vi "Main.vi"(11 "Module Admin":refnum<class "Delacor_lib_QMH_Cloneable Module Admin.lvclass">) -> ()   [LabVIEW 2023, in "VoltageDataAquisition.lvlib"]
doc: "This template is based off of the Queued Message Handler design pattern and the Queued Message Handler project template that ships with LabVIEW.\n\nThe main difference is that the queue is private to this module and communication between modules is performed via Broadcast and Request events.\n\nRequest events are wrapped in public API methods and are handled in the Event Handling Loop (EHL) of this VI. Any module can register for Broadcast events sent by this module. The EHL generates messages based on user interface actions.\n\nThe Message Handling Loop (MHL) processes messages generated by the EHL, or by other messages. The messages are string values, so new messages can be added easily to the Message Cases case structure in the MHL. Each message cluster can also provide an optional value for Message Data, which is a variant that can be converted to whatever message-specific data is required.\n_____\nBased on DQMH Project Template 7.0.1.1316."
uses:
  VoltageDataAquisition.lvlib
  <vilib>/Delacor/Delacor QMH/Libraries/Cloneable Module Admin_class/Delacor_lib_QMH_Cloneable Module Admin.lvclass
  Module Data--cluster.ctl
  <vilib>/Delacor/Delacor QMH/Libraries/Message Queue_class/Delacor_lib_QMH_Message Queue.lvclass/Delacor_lib_QMH_Message Queue.ctl
  <vilib>/Delacor/Delacor QMH/Libraries/Cloneable Module Admin_class/Delacor_lib_QMH_Cloneable Module Admin.lvclass/Delacor_lib_QMH_Cloneable Module Admin.ctl
  Stop Argument--cluster.ctl
  <vilib>/Delacor/Delacor QMH/Libraries/Module Admin_class/Delacor_lib_QMH_Module Admin.lvclass/Delacor_lib_QMH_Module Admin.ctl
  DataRead Argument--cluster.ctl
  CreatDAQ Argument--cluster.ctl
  StopDAQ Argument--cluster.ctl
  <vilib>/Utility/miscctls.llb/LVPointTypeDef.ctl
  <vilib>/Delacor/Delacor QMH/Libraries/Message Queue_class/Delacor_lib_QMH_Enqueue Message (Single).vi
  <vilib>/Delacor/Delacor QMH/Libraries/Cloneable Module Admin_class/Delacor_lib_QMH_Get Module ID.vi
  <vilib>/Delacor/Delacor QMH/Libraries/Module Admin_class/Delacor_lib_QMH_Get External Launch.vi
  <vilib>/Delacor/Delacor QMH/Libraries/Message Queue_class/Delacor_lib_QMH_Message Queue.lvclass
  <vilib>/Analysis/NI_AALBase.lvlib
panel:
  out "Stop?":bool
  out "웨이브폼 그래프":dbl[](graph)
  out "error out":errorcluster
  out "Status":string
  in  "Simulate EHL Error":bool
  in  "Simulate MHL Error":bool
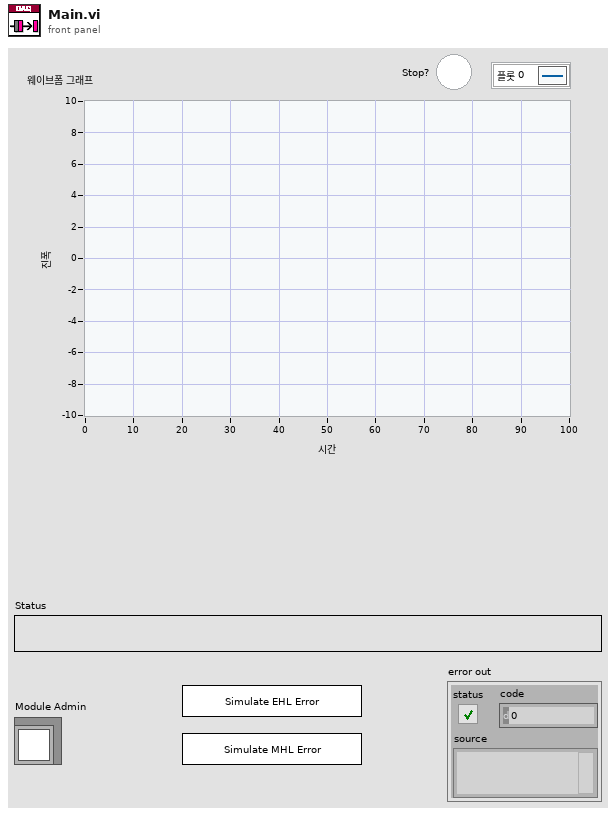
[diagram p1: front panel]
types:
  T1 = typedef "VoltageDataAquisition.lvlib/Request Events--cluster.ctl" = cluster{"Stop Module":refnum<user-event>, "Show Panel":refnum<user-event>, "Hide Panel":refnum<user-event>, "Show Diagram":refnum<user-event>, "Get Module Execution Status":refnum<user-event>, "DataRead":refnum<user-event>, "CreatDAQ":refnum<user-event>, "StopDAQ":refnum<user-event>}
  T2 = typedef "VoltageDataAquisition.lvlib/Module Data--cluster.ctl" = cluster{"Status":string, "웨이브폼 그래프":dbl[]}
  T3 = enum32{"invalid lock state", "Not Locked", "Locked (No Password)", "Password-protected"}
  T4 = typedef "VoltageDataAquisition.lvlib/Stop Argument--cluster.ctl" = cluster{"Module ID":i32, "Origin":string, "Exit via Stop Module Req?":bool, "Wait for Module to stop?":bool}
  T5 = typedef "VoltageDataAquisition.lvlib/DataRead Argument--cluster.ctl" = cluster{"Module ID":i32, "불리언":bool}
  T6 = typedef "VoltageDataAquisition.lvlib/CreatDAQ Argument--cluster.ctl" = cluster{"Module ID":i32, "불리언":bool}
  T7 = typedef "VoltageDataAquisition.lvlib/StopDAQ Argument--cluster.ctl" = cluster{"Module ID":i32, "불리언":bool}
  T8 = typedef "LVPointTypeDef.ctl" = cluster{"Horizontal":i16, "Vertical":i16}
  T9 = enum32{"Invalid", "Standard", "Closed", "Hidden", "Minimized", "Maximized"}
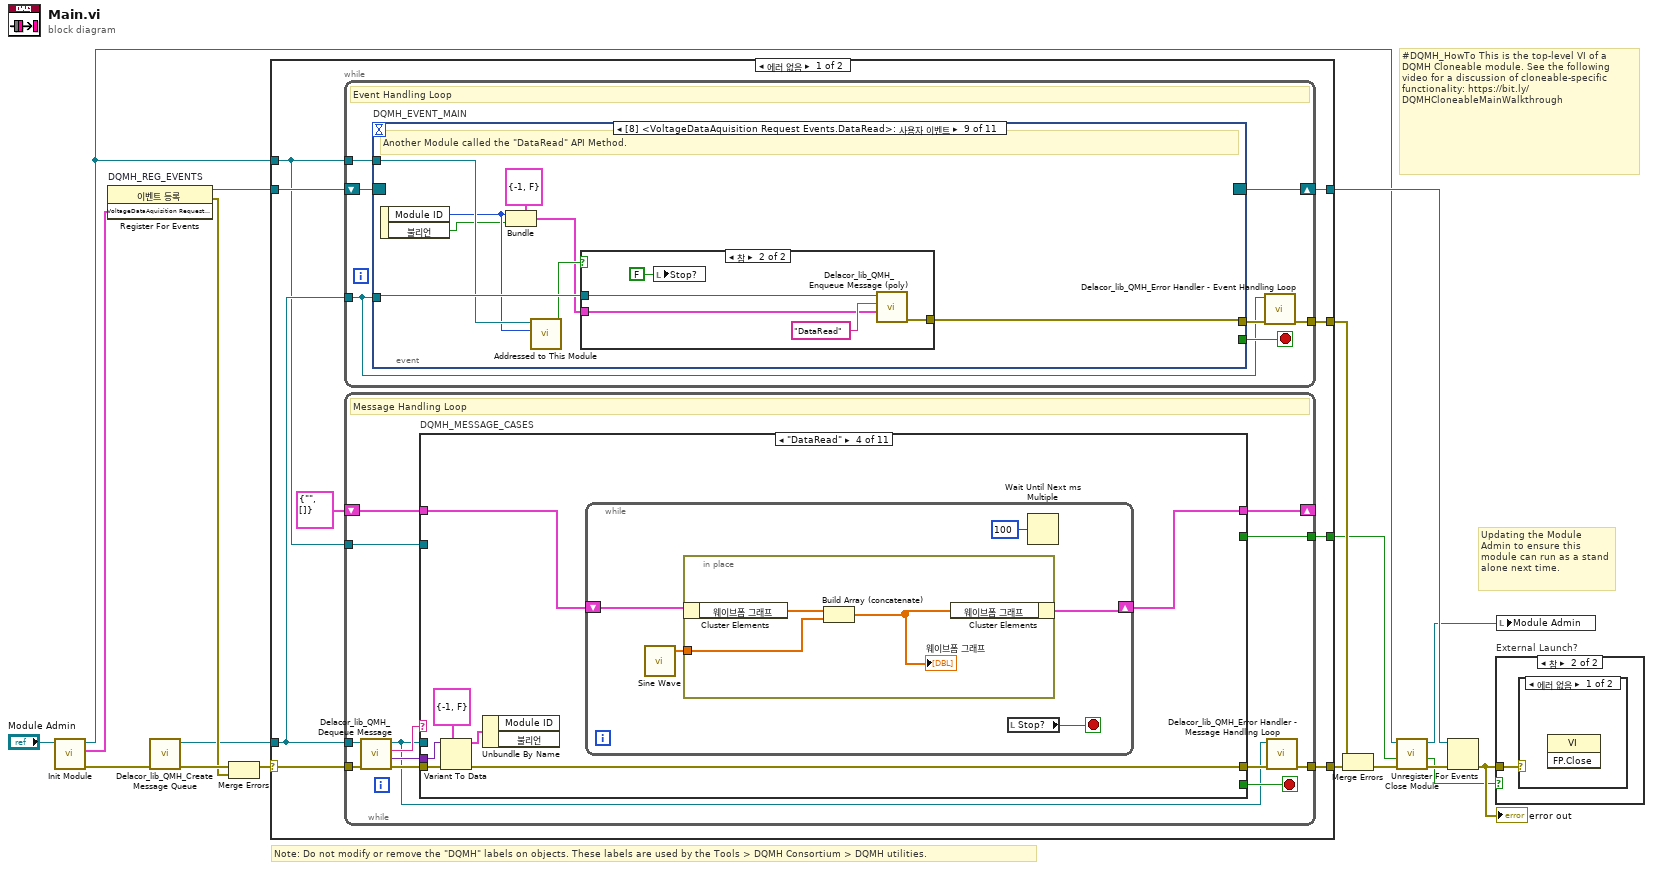
[diagram p0: block diagram]
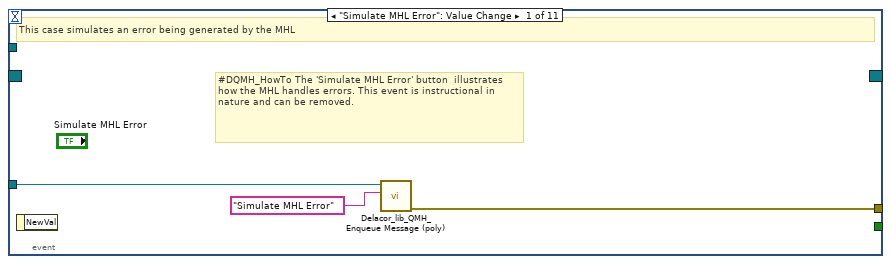
[diagram p2: hidden frame]
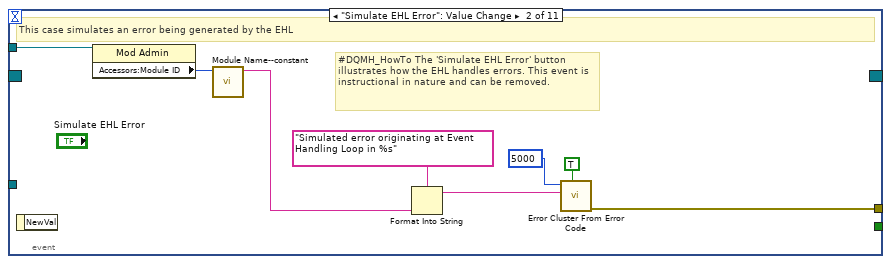
[diagram p3: hidden frame]
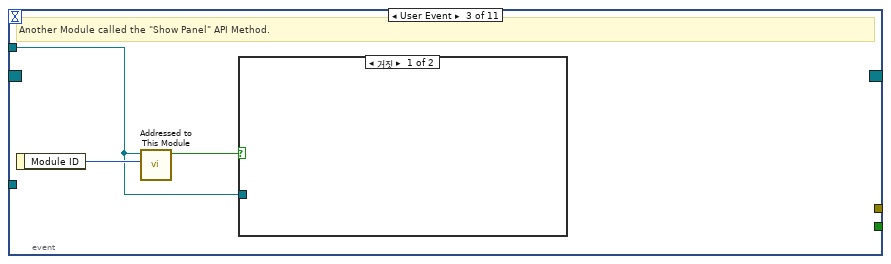
[diagram p4: hidden frame]
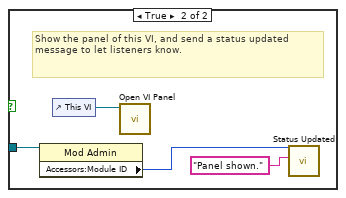
[diagram p5: hidden frame]
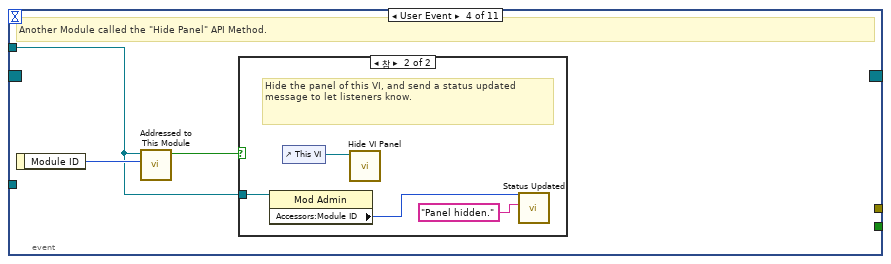
[diagram p6: hidden frame]
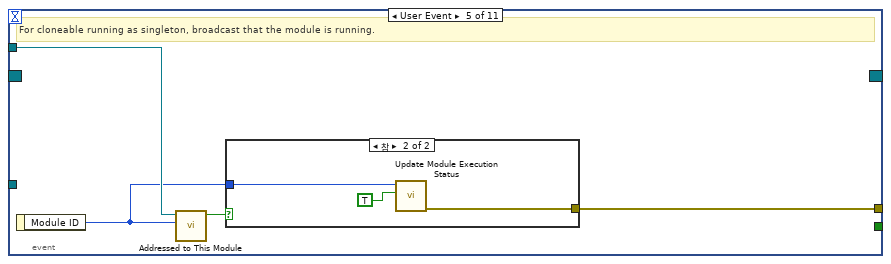
[diagram p8: hidden frame]
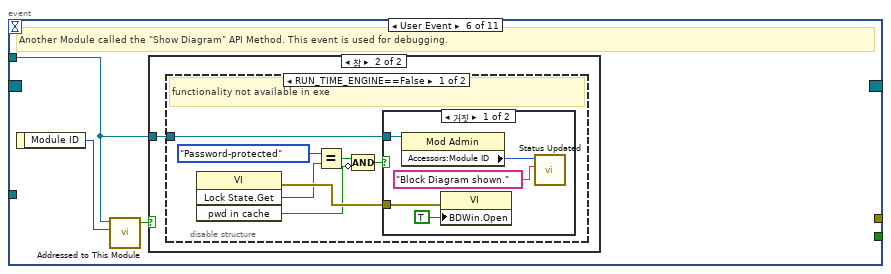
[diagram p10: hidden frame]
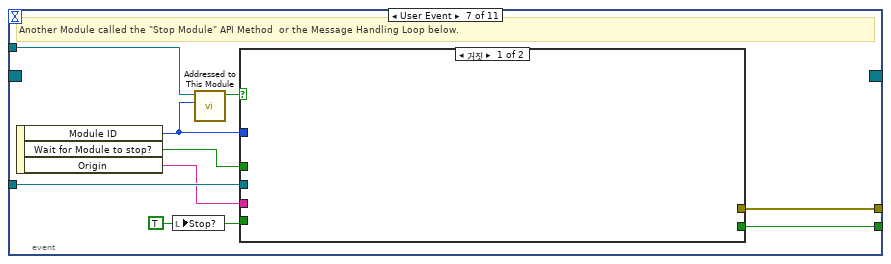
[diagram p14: hidden frame]
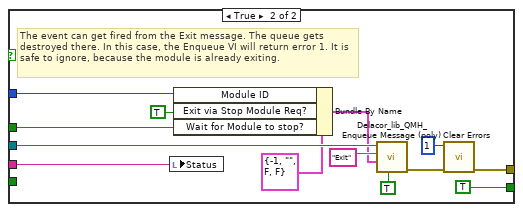
[diagram p15: hidden frame]
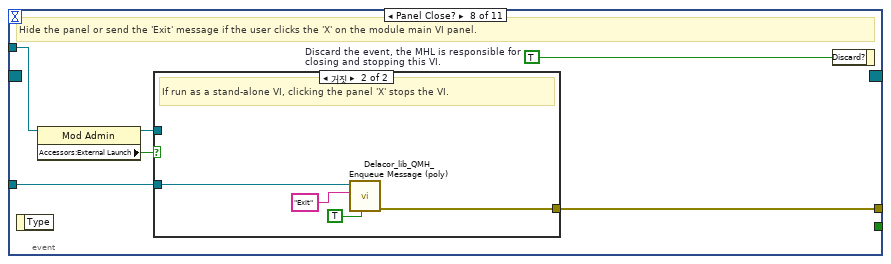
[diagram p16: hidden frame]
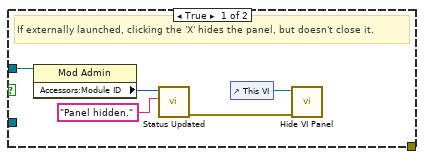
[diagram p17: hidden frame]
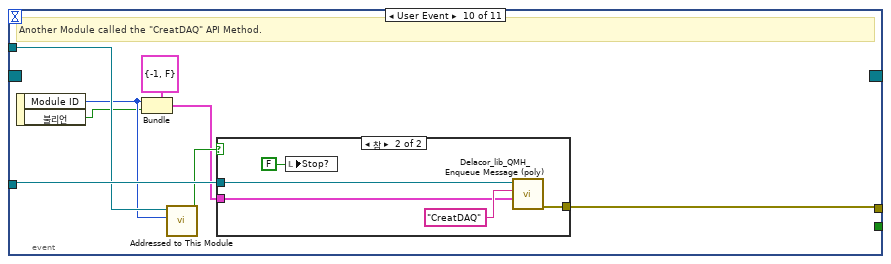
[diagram p19: hidden frame]
diagram:
  # "#DQMH_HowTo This is the top-level VI of a DQMH Cloneable module. See the following video for a discussion of cloneable-specific functionality: https://bit.ly/DQMHCloneableMainWalkthrough"
  # "Note: Do not modify or remove the \"DQMH\" labels on objects. These labels are used by the Tools > DQMH Consortium > DQMH utilities."
  # "Updating the Module Admin to ensure this module can run as a stand alone next time."
  n1 = call "Init Module.vi"("Cloneable Module Admin in"="Module Admin") -> ("error out"=w15:errorcluster, "VoltageDataAquisition Request Events"=w7:T1, "Cloneable Module Admin out"=w4:refnum<class "Delacor_lib_QMH_Cloneable Module Admin.lvclass">)  [unwired: 8 in]
  n2 = register-events "DQMH_REG_EVENTS"(w7) -> (reference out=w8:refnum<event-registration>, error out=w10:errorcluster)  [unwired: 2 in]
  n3 = call <vilib>:"Delacor_lib_QMH_Create Message Queue.vi"("error in"=w15) -> ("error out"=w12:errorcluster, "Message Queue"=w6:refnum<class "Delacor_lib_QMH_Message Queue.lvclass">)  [unwired: 9 in]
  n4 = Merge Errors(w12, w10) -> (w11:errorcluster)
  n5 = case shown="에러 없음" w11 {
    selector: w11 -> [w25 w295]
    tunnel: [w27 w294] -> w16
    tunnel: [w24 w293] -> w9
    tunnel: w8 -> [w22 w293]
    tunnel: w6 -> [w21 w286]
    tunnel: [w26 _] -> w17
    tunnel: w4 -> [w20 w289]
    tunnel: [w19 _] -> w2
    frame No Error {
      n6 = while {
        tunnel: w21 -> [w28]
        shift-right: [w31] -> w24
        shift-left: w22 -> [w32]
        tunnel: [w33] -> w26
        tunnel: w20 -> [w29]
        stop <- w30 stop-if-true
        # "Event Handling Loop"
        n7 = event "DQMH_EVENT_MAIN" shown="[8] <VoltageDataAquisition Request Events.DataRead>: 사용자 이벤트" {
          selector: w32 -> [_ _ _ _ _ _ _ _ _ _ _]
          dyn-events: [_ _ _ _ _ _ _ _ _ _ _] -> w31
          timeout: _ -> [_ _ _ _ _ _ _ _ _ _ _]
          tunnel: [_ _ _ _ _ _ w87 _ _ _ _] -> w30
          tunnel: w28 -> [w36 _ _ _ _ _ w90 w107 w127 w140 w153]
          tunnel: [w37 w45 _ _ w63 _ w91 w110 w120 w133 w146] -> w34
          tunnel: w29 -> [_ w44 w46 w53 w61 w67 w89 w108 w125 w138 w151]
          event "Simulate MHL Error": Value Change {
            # "#DQMH_HowTo The 'Simulate MHL Error' button  illustrates how the MHL handles errors. This event is instructional in nature and can be removed."
            # "This case simulates an error being generated by the MHL"
            n8 = event-data() -> ()  [unwired: 1 in, 1 out]
            n9 = call-poly <vilib>:"Delacor_lib_QMH_Enqueue Message (poly).vi"("Message"="Simulate MHL Error", "Message Queue in"=w36) -> ("error out"=w37:errorcluster)  [unwired: 8 in, 1 out]
          }
          event "Simulate EHL Error": Value Change {
            # "#DQMH_HowTo The 'Simulate EHL Error' button  illustrates how the EHL handles errors. This event is instructional in nature and can be removed."
            # "This case simulates an error being generated by the EHL"
            n10 = event-data() -> ()  [unwired: 1 in, 1 out]
            n11 = property on="Property Node" class="Mod Admin"(reference=w44) -> ("Accessors:Module ID"=w43:i32)  [unwired: 1 in, 2 out]
            n12 = call "Module Name--constant.vi"("Module ID"=w43) -> ("Module Name"=w38:string)  [unwired: 10 in]
            n13 = Format Into String(format string="Simulated error originating at Event Handling Loop in %s", w38) -> (resulting string=w41:string)  [unwired: 2 in, 1 out]
            n14 = call <vilib>:"Error Cluster From Error Code.vi"("show call chain? (False)"=TRUE, "error message (\"\")"=w41, "error code (0)"=5000) -> ("error out"=w45:errorcluster)  [unwired: 6 in]
          }
          event User Event {
            # "Another Module called the \"Show Panel\" API Method."
            n15 = event-data() -> ("Module ID"=w47:i32)  [unwired: 1 in]
            n16 = call "Addressed to This Module.vi"("Module ID from Argument"=w47, "Module Admin"=w46) -> ("Addressed to this instance?"=w48:bool)  [unwired: 8 in, 1 out]
            n17 = case shown="거짓" w48 {
              tunnel: w46 -> [_ w50]
              frame False {
              }
              frame True {
                # "Show the panel of this VI, and send a status updated message to let listeners know."
                n18 = property on="Property Node" class="Mod Admin"(reference=w50) -> ("Accessors:Module ID"=w49:i32)  [unwired: 1 in, 2 out]
                n19 = control-ref of="This VI"() -> (w52:refnum<vi>)
                n20 = call "Open VI Panel.vi"("VI"=w52) -> ()  [unwired: 10 in, 1 out]
                n21 = call "Status Updated.vi"("Status"="Panel shown." ("format string"), "Module ID"=w49) -> ()  [unwired: 9 in, 1 out]
              }
            }
          }
          event User Event {
            # "Another Module called the \"Hide Panel\" API Method."
            n22 = event-data() -> ("Module ID"=w54:i32)  [unwired: 1 in]
            n23 = call "Addressed to This Module.vi"("Module ID from Argument"=w54, "Module Admin"=w53) -> ("Addressed to this instance?"=w55:bool)  [unwired: 8 in, 1 out]
            n24 = case shown="참" w55 {
              tunnel: w53 -> [_ w57]
              frame False {
              }
              frame True {
                # "Hide the panel of this VI, and send a status updated message to let listeners know."
                n25 = property on="Property Node" class="Mod Admin"(reference=w57) -> ("Accessors:Module ID"=w56:i32)  [unwired: 1 in, 2 out]
                n26 = control-ref of="This VI"() -> (w59:refnum<vi>)
                n27 = call "Hide VI Panel.vi"("VI"=w59) -> ()  [unwired: 10 in, 1 out]
                n28 = call "Status Updated.vi"("Status"="Panel hidden." ("format string"), "Module ID"=w56) -> ()  [unwired: 9 in, 1 out]
              }
            }
          }
          event User Event {
            # "For cloneable running as singleton, broadcast that the module is running."
            n29 = event-data() -> ("Module ID"=w60:i32)  [unwired: 1 in]
            n30 = call "Addressed to This Module.vi"("Module ID from Argument"=w60, "Module Admin"=w61) -> ("Addressed to this instance?"=w62:bool)  [unwired: 8 in, 1 out]
            n31 = case shown="참" w62 {
              tunnel: [_ w66] -> w63
              tunnel: w60 -> [_ w65]
              frame False {
              }
              frame True {
                n32 = call "Update Module Execution Status.vi"("Running?"=TRUE, "Module ID"=w65) -> ("error out"=w66:errorcluster)  [unwired: 9 in]
              }
            }
          }
          event User Event {
            # "Another Module called the \"Show Diagram\" API Method. This event is used for debugging."
            n33 = event-data() -> ("Module ID"=w68:i32)  [unwired: 1 in]
            n34 = call "Addressed to This Module.vi"("Module ID from Argument"=w68, "Module Admin"=w67) -> ("Addressed to this instance?"=w69:bool)  [unwired: 8 in, 1 out]
            n35 = case shown="참" w69 {
              tunnel: w67 -> [_ w70]
              frame False {
              }
              frame True {
                n36 = disable-structure shown="RUN_TIME_ENGINE==False" {
                  disable-tunnel: w70 -> [w71 _]
                  frame condition #0 (active) {
                    # "functionality not available in exe"
                    n37 = invoke on="Invoke Node" class="VI" method="Lock State.Get"() -> (error out=w77:errorcluster, "Get Lock State"=w76:T3, "pwd in cache"=w73:bool)  [unwired: 4 in, 1 out]
                    n38 = Equal?(x=T3."Password-protected", y=w76) -> (x = y?=w74:bool)
                    n39 = Compound Arithmetic op=AND(w74, invert w73) -> (w72:bool)
                    n40 = case shown="거짓" w72 {
                      tunnel: w77 -> [w82 _]
                      tunnel: w71 -> [w79 _]
                      frame False {
                        n41 = property on="Property Node" class="Mod Admin"(reference=w79) -> ("Accessors:Module ID"=w78:i32)  [unwired: 1 in, 2 out]
                        n42 = property on="Property Node" class="VI"(error in=w82, "BDWin.Open"=TRUE ("Block Diagram Window:Open")) -> ()  [unwired: 1 in, 2 out]
                        n43 = call "Status Updated.vi"("Status"="Block Diagram shown." ("format string"), "Module ID"=w78) -> ()  [unwired: 9 in, 1 out]
                      }
                      frame True {
                        # "Password-protected VI, and the password is not in the cache. Do not show the diagram."
                      }
                    }
                  }
                  frame condition #1 {
                  }
                }
              }
            }
          }
          event User Event {
            w83 = TRUE ("Stop?")
            # "Another Module called the \"Stop Module\" API Method  or the Message Handling Loop below."
            n44 = event-data() -> ("Module ID"=w85:i32, "Wait for Module to stop?"=w86:bool, "Origin"=w84:string)  [unwired: 1 in]
            n45 = local write "Stop?"(w83) -> ()
            n46 = call "Addressed to This Module.vi"("Module ID from Argument"=w85, "Module Admin"=w89) -> ("Addressed to this instance?"=w88:bool)  [unwired: 8 in, 1 out]
            n47 = case shown="거짓" w88 {
              tunnel: [_ w103] -> w91
              tunnel: w90 -> [_ w99]
              tunnel: [_ TRUE] -> w87
              tunnel: w86 -> [_ w92]
              tunnel: w85 -> [_ w96]
              tunnel: w84 -> [_ w93]
              tunnel: w83 -> [_ _]
              frame False {
              }
              frame True {
                # "The event can get fired from the Exit message. The queue gets destroyed there. In this case, the Enqueue VI will return error 1. It is safe to ignore, because the module is already exiting."
                n48 = local write "Status"(w93) -> ()
                n49 = Bundle By Name(cluster=T4 {"Module ID"=-1, "Origin"="", "Exit via Stop Module Req?"=FALSE, "Wait for Module to stop?"=FALSE} ("Stop Argument"), "Module ID"=w96, "Exit via Stop Module Req?"=TRUE, "Wait for Module to stop?"=w92) -> (w94:T4)
                n50 = call-poly <vilib>:"Delacor_lib_QMH_Enqueue Message (poly).vi"("Priority Message? (F)"=TRUE, "Message Data"=w94, "Message"="Exit", "Message Queue in"=w99) -> ("error out"=w104:errorcluster)  [unwired: 6 in, 1 out]
                n51 = call <vilib>:"Clear Errors.vi"("error in (no error)"=w104, "specific error code to clear (0: all)"=1) -> ("error out"=w103:errorcluster)  [unwired: 4 in, 1 out]
              }
            }
          }
          event Panel Close? {
            w109 = TRUE  # Discard the event, the MHL is responsible for closing and stopping this VI.
            # "Hide the panel or send the 'Exit' message if the user clicks the 'X' on the module main VI panel."
            n52 = event-data() -> ()  [unwired: 1 in, 1 out]
            n53 = property on="Property Node" class="Mod Admin"(reference=w108) -> (reference out=w105:refnum<class "Delacor_lib_QMH_Cloneable Module Admin.lvclass">, "Accessors:External Launch"=w106:bool)  [unwired: 1 in, 1 out]
            n54 = case shown="거짓" w106 {
              tunnel: w107 -> [_ w118]
              tunnel: [_ w119] -> w110
              tunnel: w105 -> [w113 _]
              frame True {
                # "If externally launched, clicking the 'X' hides the panel, but doesn't close it."
                n55 = property on="Property Node" class="Mod Admin"(reference=w113) -> ("Accessors:Module ID"=w112:i32)  [unwired: 1 in, 2 out]
                n56 = call "Status Updated.vi"("Status"="Panel hidden." ("format string"), "Module ID"=w112) -> ("error out"=w111:errorcluster)  [unwired: 9 in]
                n57 = control-ref of="This VI"() -> (w115:refnum<vi>)
                n58 = call "Hide VI Panel.vi"("error in"=w111, "VI"=w115) -> ()  [unwired: 9 in, 1 out]
              }
              frame False {
                # "If run as a stand-alone VI, clicking the panel 'X' stops the VI."
                n59 = call-poly <vilib>:"Delacor_lib_QMH_Enqueue Message (poly).vi"("Priority Message? (F)"=TRUE, "Message"="Exit", "Message Queue in"=w118) -> ("error out"=w119:errorcluster)  [unwired: 7 in, 1 out]
              }
            }
            n60 = event-data ("Event Filter Node")("Discard?"=w109) -> ()  [unwired: 1 in, 1 out]
          }
          event User Event {
            # "Another Module called the \"DataRead\" API Method."
            n61 = event-data() -> ("Module ID"=w122:i32, "불리언"=w121:bool)  [unwired: 1 in]
            n62 = Bundle(cluster=T5 {"Module ID"=-1, "불리언"=FALSE} ("DataRead Argument"), "Module ID"=w122, "불리언"=w121) -> (w123:T5)
            n63 = call "Addressed to This Module.vi"("Module ID from Argument"=w122, "Module Admin"=w125) -> ("Addressed to this instance?"=w126:bool)  [unwired: 8 in, 1 out]
            n64 = case "케이스 구조" shown="참" w126 {
              tunnel: w127 -> [_ w132]
              tunnel: w123 -> [_ w130]
              tunnel: [_ w129] -> w120
              frame False {
              }
              frame True {
                n65 = local write "Stop?"(FALSE ("Stop?")) -> ()
                n66 = call-poly <vilib>:"Delacor_lib_QMH_Enqueue Message (poly).vi"("Message Data"=w130, "Message"="DataRead", "Message Queue in"=w132) -> ("error out"=w129:errorcluster)  [unwired: 7 in, 1 out]
              }
            }
          }
          event User Event {
            # "Another Module called the \"CreatDAQ\" API Method."
            n67 = event-data() -> ("Module ID"=w135:i32, "불리언"=w134:bool)  [unwired: 1 in]
            n68 = Bundle(cluster=T6 {"Module ID"=-1, "불리언"=FALSE} ("CreatDAQ Argument"), "Module ID"=w135, "불리언"=w134) -> (w136:T6)
            n69 = call "Addressed to This Module.vi"("Module ID from Argument"=w135, "Module Admin"=w138) -> ("Addressed to this instance?"=w139:bool)  [unwired: 8 in, 1 out]
            n70 = case "케이스 구조" shown="참" w139 {
              tunnel: w140 -> [_ w145]
              tunnel: w136 -> [_ w143]
              tunnel: [_ w142] -> w133
              frame False {
              }
              frame True {
                n71 = local write "Stop?"(FALSE ("Stop?")) -> ()
                n72 = call-poly <vilib>:"Delacor_lib_QMH_Enqueue Message (poly).vi"("Message Data"=w143, "Message"="CreatDAQ", "Message Queue in"=w145) -> ("error out"=w142:errorcluster)  [unwired: 7 in, 1 out]
              }
            }
          }
          event User Event {
            # "Another Module called the \"StopDAQ\" API Method."
            n73 = event-data() -> ("Module ID"=w148:i32, "불리언"=w147:bool)  [unwired: 1 in]
            n74 = Bundle(cluster=T7 {"Module ID"=-1, "불리언"=FALSE} ("StopDAQ Argument"), "Module ID"=w148, "불리언"=w147) -> (w149:T7)
            n75 = call "Addressed to This Module.vi"("Module ID from Argument"=w148, "Module Admin"=w151) -> ("Addressed to this instance?"=w152:bool)  [unwired: 8 in, 1 out]
            "Stop?" <- w152
            n76 = case "케이스 구조" shown="참" w152 {
              tunnel: w153 -> [_ w157]
              tunnel: w149 -> [_ w155]
              tunnel: [_ w154] -> w146
              frame False {
              }
              frame True {
                n77 = call-poly <vilib>:"Delacor_lib_QMH_Enqueue Message (poly).vi"("Message Data"=w155, "Message"="StopDAQ", "Message Queue in"=w157) -> ("error out"=w154:errorcluster)  [unwired: 7 in, 1 out]
              }
            }
          }
        }
        n78 = call-dynamic "Delacor_lib_QMH_Error Handler - Event Handling Loop.vi"("error in"=w34, "Message Queue in"=w28) -> ("dup error in"=w33:errorcluster)  [unwired: 8 in, 1 out]
      }
      n79 = while {
        tunnel: w21 -> [w158]
        shift-right: [w165] -> _
        shift-left: T2 {"Status"="", "웨이브폼 그래프"=[]} ("Data Cluster") -> [w166]
        tunnel: w25 -> [w169]
        tunnel: [w167] -> w27
        tunnel: w20 -> [w160]
        tunnel: [w159] -> w19
        stop <- w164 stop-if-true
        # "Message Handling Loop"
        n80 = call-dynamic "Delacor_lib_QMH_Dequeue Message.vi"("error in"=w169, "Message Queue in"=w158) -> ("error out"=w168:errorcluster, "Message Data"=w162:variant, "Message"=w163:string, "Message Queue out"=w161:refnum<class "Delacor_lib_QMH_Message Queue.lvclass">)  [unwired: 6 in]
        n81 = case "DQMH_MESSAGE_CASES" shown="\"DataRead\"" w163 {
          selector: w163 -> [_ _ _ _ _ _ _ _ _ _ w275]
          tunnel: w161 -> [_ _ _ _ _ _ _ w230 _ w267 _]
          tunnel: w168 -> [w189 w193 w200 w208 w222 w225 w227 w239 w256 w273 w284]
          tunnel: [w187 w193 w199 w207 w220 w224 w227 w235 w255 w268 w285] -> w170
          tunnel: w166 -> [w180 w192 w195 w203 w221 w223 w226 w234 w253 w266 w282]
          tunnel: [w179 w192 w194 w202 w221 w223 w226 w234 w253 w266 w282] -> w165
          tunnel: [_ _ _ _ _ _ _ _ _ w265 _] -> w164
          tunnel: w162 -> [_ _ w198 w206 w219 _ _ w233 _ w263 _]
          tunnel: w160 -> [w174 _ _ _ _ _ _ w232 w251 w258 w281]
          tunnel: [_ _ _ _ _ _ _ _ _ w261 _] -> w159
          frame "Initialize" {
            w171 = "Initial Message" ("Initial Message")
            # "#CodeNeeded - Initialize the appearance of the front panel."
            # "#CodeNeeded - Initialize your state data here."
            # "Initialize - Any operation that needs to be done before the module can receive messages. Synchronize Caller Events.vi will inform Start Module.vi that the module has launched and is ready to receive messages. Module Did Init.vi will broadcast that the module initialized."
            n82 = call "Synchronize Caller Events.vi"("error in"=w189, "Module Admin"=w174) -> ("error out"=w188:errorcluster, "Module Admin out"=w173:refnum<class "Delacor_lib_QMH_Cloneable Module Admin.lvclass">)  [unwired: 8 in]
            n83 = property on="Property Node" class="Mod Admin"(reference=w173) -> ("Accessors:Module ID"=w176:i32, "Accessors:External Launch"=w175:bool)  [unwired: 1 in, 2 out]
            n84 = call "Module Name--constant.vi"("Module ID"=w176) -> ("Module Name"=w184:string)  [unwired: 10 in]
            n85 = property on="Property Node" class="VI"("Front Panel.Title"=w184) -> (reference out=w186:refnum<vi>, error out=w191:errorcluster)  [unwired: 2 in]
            n86 = Select(t=T9."Hidden" ("State"), s=w175, f=T9."Standard" ("State")) -> (s? t:f=w181:T9)
            n87 = invoke on="Invoke Node" class="VI" method="FP.Open"(reference=w186, error in=w191, "State"=w181) -> (reference out=w185:refnum<vi>, error out=w190:errorcluster)  [unwired: 2 in, 3 out]
            n88 = call "Module Name--constant.vi"("Module ID"=w176) -> ("Module Name"=w177:string)  [unwired: 10 in]
            n89 = Bundle By Name(cluster=w180, "Status"=w171) -> (w179:T2)
            n90 = invoke on="Invoke Node" class="VI" method="FP.Center"(reference=w185, error in=w190) -> ()  [unwired: 1 in, 3 out]
            n91 = property on="Pane" class="Pane"("Origin"=T8 {"Horizontal"=0, "Vertical"=0}) -> ()  [unwired: 2 in, 2 out]
            n92 = call "Module Did Init.vi"("error in"=w188, "Initialized?"=TRUE, "Origin"=w177, "Module ID"=w176) -> ("error out"=w187:errorcluster)  [unwired: 7 in]
            "Status" <- w171
          }
          frame "---Module Specific---" {
            # "Separator -- The following cases handle messages specific to this Module."
          }
          frame "CreatDAQ" {
            n93 = Variant To Data(error in=w200, type=T6 {"Module ID"=-1, "불리언"=FALSE} ("CreatDAQ Argument"), Variant=w198) -> (data=w196:T6, error out=w199:errorcluster)
            n94 = Unbundle By Name(w196) -> ()  [unwired: 2 out]
            n95 = in-place {
              n96 = in-place-cluster #1(w195) -> ()  [unwired: 1 out]
              n97 = in-place-cluster #1("웨이브폼 그래프"=dbl[] [] ("웨이브폼 차트")) -> (w194:T2)
            }
          }
          frame "DataRead" {
            n98 = Variant To Data(error in=w208, type=T5 {"Module ID"=-1, "불리언"=FALSE} ("DataRead Argument"), Variant=w206) -> (data=w204:T5, error out=w207:errorcluster)
            n99 = Unbundle By Name(w204) -> ()  [unwired: 2 out]
            n100 = while {
              shift-right: [w212] -> w202
              shift-left: w203 -> [w213]
              stop <- w211 stop-if-true
              n101 = call <vilib>:"Sine Wave.vi"() -> ("sine wave"=w209:dbl[])  [unwired: 5 in, 2 out]
              n102 = in-place {
                in-place-border: w209 -> [w215]
                n103 = in-place-cluster #2(w213) -> ("웨이브폼 그래프"=w216:dbl[])
                n104 = Build Array (concatenate)(w216, w215) -> (w214:dbl[])
                "웨이브폼 그래프" <- w214
                n105 = in-place-cluster #2("웨이브폼 그래프"=w214) -> (w212:T2)
              }
              n106 = local read "Stop?"() -> (w211:bool)
              n107 = Wait Until Next ms Multiple(millisecond multiple=u32 100 ("ms 배수")) -> ()  [unwired: 1 out]
            }
          }
          frame "StopDAQ" {
            n108 = Variant To Data(error in=w222, type=T7 {"Module ID"=-1, "불리언"=FALSE} ("StopDAQ Argument"), Variant=w219) -> (data=w217:T7, error out=w220:errorcluster)
            n109 = Unbundle By Name(w217) -> ()  [unwired: 2 out]
          }
          frame "---Copy This Frame---" {
            # "Duplicate this frame when creating new messages.  Change this comment in the duplicated frame to describe this message."
            n110 = Merge Errors(w225) -> (w224:errorcluster)
          }
          frame "---Exit and Error Handling---" {
            # "Separator - the following cases handle errors and exit messages."
          }
          frame "Error" {
            # "#CodeRecommended - If the module is running in standalone mode (External Launch = FALSE), this code will pop up an error dialog and call the 'Exit' message if an error occurs. Add more fine-grained error management here."
            # "Error - Check the error message data and respond accordingly. This message is sent by the \"Error Handler\" VIs at the end of each loop in this application."
            n111 = property on="Property Node" class="Mod Admin"(reference=w232) -> ("Accessors:External Launch"=w231:bool, "Accessors:Module ID"=w229:i32)  [unwired: 1 in, 2 out]
            n112 = Variant To Data(error in=w239, type=errorcluster {"status"=FALSE, "code"=0, "source"=""} ("error constant"), Variant=w233) -> (data=w228:errorcluster, error out=w237:errorcluster)
            n113 = local write "error out"(w228) -> ()
            n114 = call "Error Reported.vi"("Error"=w228, "Module ID"=w229) -> ()  [unwired: 9 in, 1 out]
            n115 = case shown="거짓" w231 {
              tunnel: [w244 _] -> w236
              tunnel: w230 -> [w242 _]
              tunnel: w228 -> [w243 _]
              frame False {
                n116 = disable-structure shown="Default" {
                  disable-tunnel: w243 -> [w245 _]
                  frame condition #0 (active) {
                    # "If the module is running standalone, then pop up an error dialog and call the \"Exit\" message."
                    n117 = call <vilib>:"Simple Error Handler.vi"("error in (no error)"=w245) -> ()  [unwired: 4 in, 5 out]
                  }
                  frame condition #1 {
                    # "To prevent the Simple Error Handler VI from being loaded (e.g. when deploying to a Real-Time target), add the Conditional Disable Symbol \"DQMH_Disable_SEH\" to your project and set it to TRUE."
                  }
                }
                n118 = call-poly <vilib>:"Delacor_lib_QMH_Enqueue Message (poly).vi"("Priority Message? (F)"=TRUE, "Message"="Exit", "Message Queue in"=w242) -> ("error out"=w244:errorcluster)  [unwired: 7 in, 1 out]
              }
              frame True {
                # "If the module was launched externally, calling the Error Reported broadcast VI is the only action performed by the \"Error\" message. The module's caller can then process the error appropriately."
              }
            }
            n119 = Merge Errors(w237, w236) -> (w235:errorcluster)
          }
          frame "Simulate MHL Error" {
            # "#DQMH_HowTo The 'Simulate MHL Error' button  illustrates how the MHL handles errors. This event is instructional in nature and can be removed."
            # "Simulate an error occurring at the MHL"
            n120 = property on="Property Node" class="Mod Admin"(reference=w251) -> ("Accessors:Module ID"=w252:i32)  [unwired: 1 in, 2 out]
            n121 = call "Module Name--constant.vi"("Module ID"=w252) -> ("Module Name"=w247:string)  [unwired: 10 in]
            n122 = Format Into String(format string="Simulated error originating at Message Handling Loop in %s", w247) -> (resulting string=w248:string)  [unwired: 2 in, 1 out]
            n123 = call <vilib>:"Error Cluster From Error Code.vi"("show call chain? (False)"=TRUE, "error message (\"\")"=w248, "error code (0)"=5001) -> ("error out"=w254:errorcluster)  [unwired: 6 in]
            n124 = Merge Errors(w256, w254) -> (w255:errorcluster)
          }
          frame "Exit" {
            w264 = 91  # 91: not all Exit messages will have an argument
            w265 = TRUE  # Stop the VI
            # "Release the message queue reference"
            # "#CodeNeeded - Add any required cleanup code here."
            # "Exit - Exit the application."
            n125 = Variant To Data(error in=w273, type=T4 {"Module ID"=-1, "Origin"="", "Exit via Stop Module Req?"=FALSE, "Wait for Module to stop?"=FALSE} ("Stop Argument"), Variant=w263) -> (data=w260:T4, error out=w269:errorcluster)
            n126 = call <vilib>:"Clear Errors.vi"("error in (no error)"=w269, "specific error code to clear (0: all)"=w264) -> ("error out"=w272:errorcluster)  [unwired: 4 in, 1 out]
            n127 = property on="Property Node" class="Mod Admin"(reference=w258) -> ("Accessors:Module ID"=w257:i32)  [unwired: 1 in, 2 out]
            n128 = control-ref of="This VI"() -> (w259:refnum<vi>)
            n129 = call-dynamic "Delacor_lib_QMH_Release Message Queue.vi"("error in"=w272, "Message Queue"=w267) -> ("error out"=w271:errorcluster)  [unwired: 9 in]
            n130 = call "Handle Exit.vi"("Stop Argument"=w260, "Module Admin in"=w258, "VI reference"=w259) -> ("error out"=w270:errorcluster, "Wait for Stop?"=w261:bool)  [unwired: 7 in]
            n131 = Merge Errors(w271, w270) -> (w268:errorcluster)
            n132 = call "Error Reported.vi"("Error"=w268, "Module ID"=w257) -> ()  [unwired: 9 in, 1 out]
          }
          frame Default {
            # "'Default' case only runs if there is a message that isn't defined in any of the other cases.  Output a programming error."
            n133 = property on="Property Node" class="Mod Admin"(reference=w281) -> ("Accessors:Module ID"=w280:i32)  [unwired: 1 in, 2 out]
            n134 = call "Module Name--constant.vi"("Module ID"=w280) -> ("Module Name"=w274:string)  [unwired: 10 in]
            n135 = Format Into String(format string="The invalid message string \"%s\" was received in the Message Handling Loop for module \"%s\".", w275, w274) -> (resulting string=w277:string)  [unwired: 2 in, 1 out]
            n136 = call <vilib>:"Error Cluster From Error Code.vi"("show call chain? (False)"=TRUE, "error message (\"\")"=w277, "error code (0)"=1) -> ("error out"=w283:errorcluster)  [unwired: 6 in]
            n137 = Merge Errors(w284, w283) -> (w285:errorcluster)
          }
        }
        n138 = call-dynamic "Delacor_lib_QMH_Error Handler - Message Handling Loop.vi"("error in"=w170, "Message Queue in"=w161) -> ("dup error in"=w167:errorcluster)  [unwired: 8 in, 1 out]
      }
    }
    frame Error {
      n139 = call "Synchronize Caller Events.vi"("Module Admin"=w289) -> ("Module Admin out"=w288:refnum<class "Delacor_lib_QMH_Cloneable Module Admin.lvclass">)  [unwired: 9 in, 1 out]
      n140 = property on="Property Node" class="Mod Admin"(reference=w288) -> ("Accessors:Module ID"=w287:i32)  [unwired: 1 in, 2 out]
      n141 = call-dynamic "Delacor_lib_QMH_Release Message Queue.vi"("error in"=w295, "Message Queue"=w286) -> ("error out"=w294:errorcluster)  [unwired: 9 in]
      n142 = call "Module Name--constant.vi"("Module ID"=w287) -> ("Module Name"=w292:string)  [unwired: 10 in]
      n143 = Format Into String(format string="An error occurred during initialization. %s is no longer running.", w292) -> (resulting string=w290:string)  [unwired: 2 in, 1 out]
      n144 = call "Error Reported.vi"("Additional Information"=w290, "Error"=w294, "Module ID"=w287) -> ()  [unwired: 8 in, 1 out]
    }
  }
  n145 = Merge Errors(w17, w16) -> (w18:errorcluster)
  n146 = call "Close Module.vi"("error in"=w18, "Wait for stop?"=w2, "Module Admin in"=w4) -> ("error out"=w14:errorcluster, "External Launch"=w1:bool, "Module Admin out"=w3:refnum<class "Delacor_lib_QMH_Cloneable Module Admin.lvclass">)  [unwired: 6 in]
  n147 = Unregister For Events(event registration refnum=w9, error in=w14) -> (error out=w13:errorcluster)
  "error out" <- w13
  n148 = case "External Launch?" shown="참" w1 {
    tunnel: w13 -> [_ w296]
    frame False {
    }
    frame True {
      n149 = case shown="에러 없음" w296 {
        frame No Error {
          n150 = invoke class="VI" method="FP.Close"() -> ()  [unwired: 3 in, 3 out]
        }
        frame Error {
          n151 = invoke class="VI" method="FP.Open"("Activate"=TRUE ("Activate?")) -> ()  [unwired: 4 in, 5 out]
        }
      }
    }
  }
  n152 = local write "Module Admin"(w3) -> ()
